vi "Add PV (String).vi"(5 "is read only? (F)":bool, 6 "initial timestamp":timestamp, 7 "PV name":string, 8 "error in (no error)":errorcluster, 10 "initial value":string, 11 "Server in":refnum<class "Server.lvclass">) -> (0 "error out":errorcluster, 2 "value out":string, 3 "Server out":refnum<class "Server.lvclass">, 4 "timestamp out":timestamp)   [LabVIEW 2020, in "PV Access.lvlib" / "PVA Server.lvlib" / "Server.lvclass"]
uses:
  Server.lvclass
  PV Data/NT Scalar/NT Scalar.lvclass
  C:/Users/eyw68381/source/repos/pvaccess-labview/labview/source/PV Data/NT Base/NT Base.lvclass
  Server.lvclass/Server.ctl
  Source/Source.lvclass
  PV Data/PV Data.lvlib
  PV Data/NT Scalar/Create (String).vi
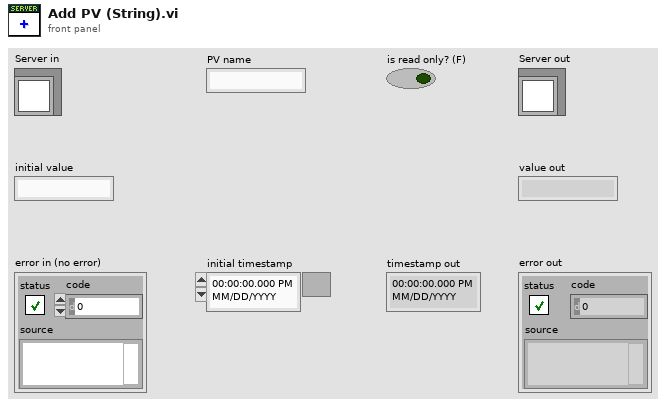
[diagram p1: front panel]
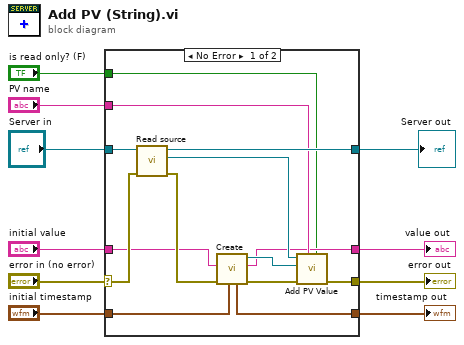
[diagram p0: block diagram]
diagram:
  n1 = case shown="No Error" "error in (no error)" {
    selector: "error in (no error)" -> [w20 w28]
    tunnel: [w19 w28] -> w9
    tunnel: [w23 w27] -> w7
    tunnel: "Server in" -> [w24 w27]
    tunnel: "PV name" -> [w21 _]
    tunnel: "initial value" -> [w15 w26]
    tunnel: [w14 w26] -> w4
    tunnel: "initial timestamp" -> [w13 w25]
    tunnel: [w12 w25] -> w2
    tunnel: "is read only? (F)" -> [w11 _]
    frame No Error {
      n2 = call "Read source.vi"("error in (no error)"=w20, "Server in"=w24) -> ("error out"=w18:errorcluster, "Source"=w22:refnum<class "Source.lvclass">, "Server out"=w23:refnum<class "Server.lvclass">)  [unwired: 7 in]
      n3 = call-poly "Create.vi"("timestamp in"=w13, "error in (no error)"=w18, "value in"=w15) -> ("error out"=w17:errorcluster, "value out"=w14:string, "NT Scalar out"=w16:refnum<class "NT Scalar.lvclass">, "timestamp out"=w12:timestamp)  [unwired: 5 in]
      n4 = call "Add PV Value.vi"("is read only? (F)"=w11, "PV name"=w21, "error in"=w17, "NT Base in"=w16, "Source in"=w22) -> ("error out"=w19:errorcluster)  [unwired: 4 in, 2 out]
    }
    frame Error {
    }
  }
  "error out" <- w9
  "Server out" <- w7
  "value out" <- w4
  "timestamp out" <- w2
